vi "SvgDoc Save As Emf.vi"(8 "error in (no error)":errorcluster, 10 "Emf Path":path, 11 "SVG DOC":refnum<k24>) -> (0 "error out":errorcluster, 3 "SVG DOC out":refnum<k24>)   [LabVIEW 2020, in "SvgDotNet.lvlib"]
uses:
  SvgDotNet.lvlib
  C:/Users/huipeng8/Desktop/SVG.NET/Svg.dll
  Svg.dll
  System.Drawing
panel:
  # "Connector Pane"
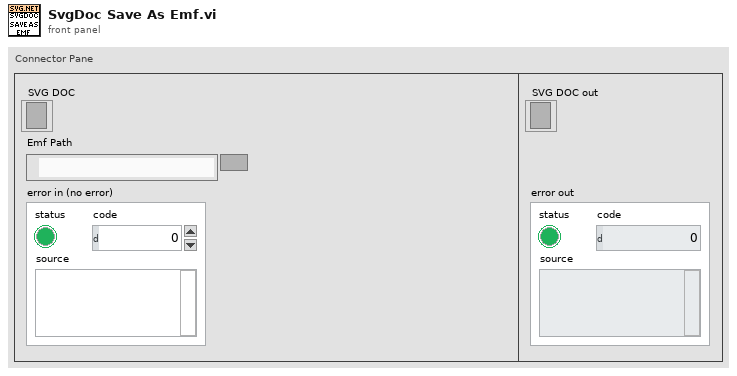
[diagram p1: front panel]
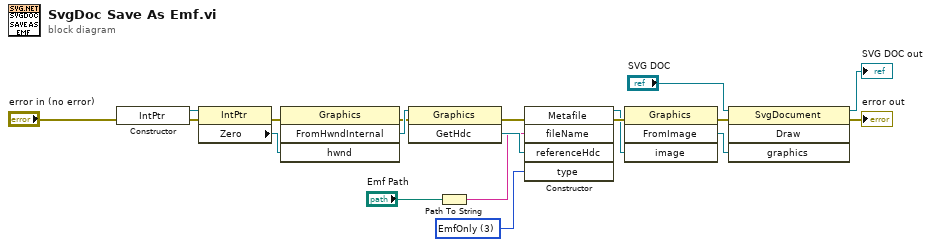
[diagram p0: block diagram]
diagram:
  w10 = 3 items=["EmfOnly"=3, "EmfPlusOnly"=4, "EmfPlusDual"=5] ("type")
  n1 = constructor class="IntPtr"(error in="error in (no error)") -> (reference out=w14:refnum<k24>, error out=w15:errorcluster)  [unwired: 2 in, 1 out]
  n2 = property class="IntPtr"(reference=w14, error in=w15) -> (error out=w16:errorcluster, "Zero"=w13:refnum<k24>)  [unwired: 1 out]
  n3 = invoke class="Graphics" method="FromHwndInternal"(error in=w16, "hwnd"=w13) -> (error out=w7:errorcluster, "FromHwndInternal"=w11:refnum<k24>)  [unwired: 2 in, 2 out]
  n4 = invoke class="Graphics" method="GetHdc"(reference=w11, error in=w7) -> (error out=w8:errorcluster, "GetHdc"=w5:refnum<k24>)  [unwired: 1 in, 1 out]
  n5 = Path To String(path="Emf Path") -> (string=w4:string)
  n6 = constructor class="Metafile"(error in=w8, "fileName"=w4, "referenceHdc"=w5, "type"=w10) -> (reference out=w6:refnum<k24>, error out=w9:errorcluster)  [unwired: 2 in, 4 out]
  n7 = invoke class="Graphics" method="FromImage"(error in=w9, "image"=w6) -> (error out=w2:errorcluster, "FromImage"=w12:refnum<k24>)  [unwired: 2 in, 2 out]
  n8 = invoke class="SvgDocument" method="Draw"(reference="SVG DOC", error in=w2, "graphics"=w12) -> (reference out=→"SVG DOC out":refnum<k24>, error out=→"error out":errorcluster)  [unwired: 1 in, 2 out]
